vi "4motors.vi"(6 "Reset":bool, 8 "error in (no error)":errorcluster, 9 "dt(s)":dbl=-1.0 format="%.3f", 11 "Power":dbl[](array[numeric])) -> (0 "error out":errorcluster, 3 "Encorder":dbl[](array[numeric]))   [LabVIEW 2018]
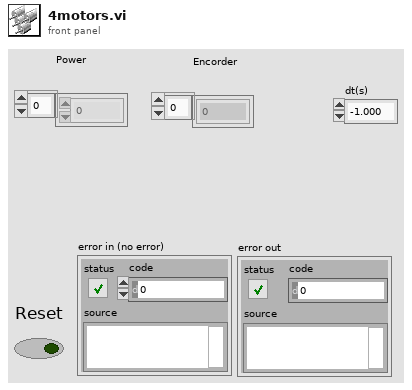
[diagram p1: front panel]
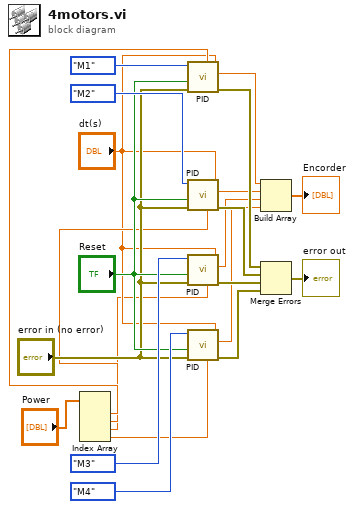
[diagram p0: block diagram]
diagram:
  n1 = Index Array(array="Power") -> (element #1=w8:dbl, element #2=w7:dbl, element #3=w1:dbl, element #4=w6:dbl)  [unwired: 4 in]
  n2 = call "PID.vi"("dt(s)"="dt(s)", "s"=w8, "error in (no error)"="error in (no error)", "Reset"="Reset", "Enum"=enum16{"M4", "M3", "M2", "M1"}."M1") -> ("error out 2"=w13:errorcluster, "en/deg"=w4:dbl)  [unwired: 3 in]
  n3 = call "PID.vi"("dt(s)"="dt(s)", "s"=w7, "error in (no error)"="error in (no error)", "Reset"="Reset", "Enum"=enum16{"M4", "M3", "M2", "M1"}."M2") -> ("error out 2"=w14:errorcluster, "en/deg"=w9:dbl)  [unwired: 3 in]
  n4 = call "PID.vi"("dt(s)"="dt(s)", "s"=w1, "error in (no error)"="error in (no error)", "Reset"="Reset", "Enum"=enum16{"M4", "M3", "M2", "M1"}."M3") -> ("error out 2"=w15:errorcluster, "en/deg"=w10:dbl)  [unwired: 3 in]
  n5 = call "PID.vi"("dt(s)"="dt(s)", "s"=w6, "error in (no error)"="error in (no error)", "Reset"="Reset", "Enum"=enum16{"M4", "M3", "M2", "M1"}."M4") -> ("error out 2"=w16:errorcluster, "en/deg"=w3:dbl)  [unwired: 3 in]
  n6 = Build Array(w4, w9, w10, w3) -> (→"Encorder":dbl[])
  n7 = Merge Errors(w13, w14, w15, w16) -> (→"error out":errorcluster)
